vi "Msg.vi"(7 "jettl in":refnum<class "jettl.lvclass">, 11 "Template Msg Strategy in":refnum<class "Template Msg Strategy.lvclass">) -> (5 "jettl out":refnum<class "jettl.lvclass">)   [LabVIEW 2021, in "_Refactor Msg.lvlib" / "jettl Msg Template.lvlib" / "Template Msg Strategy.lvclass"]
uses:
  Template Msg Strategy.lvclass
  _Template/Templates/jettl Msg Template/jettl Msg Template/jettl Msg Template.lvclass
  <vilib>/jettl/jettl/jettl/jettl/jettl.lvclass
  C:/git/jettl/tools/Template/_Refactor Msg/Template/Template Msg Strategy/Template Msg Strategy.lvclass
  C:/Program Files/National Instruments/LabVIEW 2021/vi.lib/jettl/jettl/jettl/Msg Strategy/Msg Strategy.lvclass
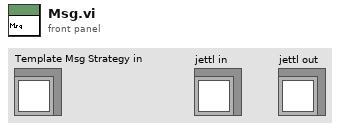
[diagram p1: front panel]
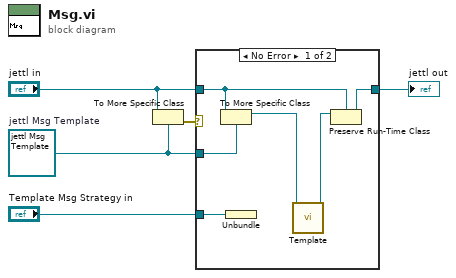
[diagram p0: block diagram]
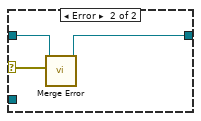
[diagram p2: hidden frame]
diagram:
  w2 = refnum<class "jettl Msg Template.lvclass"> refnum  # jettl Msg Template
  n1 = To More Specific Class(target class=w2, reference="jettl in") -> (error out=w5:errorcluster)  [unwired: 1 in, 1 out]
  n2 = case shown="No Error" w5 {
    selector: w5 -> [_ w13]
    tunnel: [w9 w12] -> w3
    tunnel: "jettl in" -> [w10 w14]
    tunnel: w2 -> [w11 _]
    tunnel: "Template Msg Strategy in" -> [w6 _]
    frame No Error {
      n3 = To More Specific Class(target class=w11, reference=w10) -> (specific class reference=w8:refnum<class "jettl Msg Template.lvclass">)  [unwired: 1 in, 1 out]
      n4 = Unbundle "Unbundle"(w6) -> ()  [unwired: 1 out]
      n5 = call-dynamic "Template.vi"("jettl Msg Template in"=w8) -> ("jettl Msg Template out"=w7:refnum<class "jettl Msg Template.lvclass">)  [unwired: 10 in]
      n6 = Preserve Run-Time Class(object in=w7, 2:w10) -> (object out=w9:refnum<class "jettl.lvclass">)  [unwired: 1 in, 1 out]
    }
    frame Error {
      n7 = call-dynamic "Merge Error.vi"("Error"=w13, "jettl Msg Merge Error in"=w14) -> ("jettl Msg Merge Error out"=w12:refnum<class "jettl.lvclass">)  [unwired: 9 in]
    }
  }
  "jettl out" <- w3
